vi "getVersion.vi"(8 "error in (no error)":errorcluster) -> (0 "error out":errorcluster, 2 "sbgComVersion":string, 3 "sbgMatLabVersion":string)   [LabVIEW 2011, in "sbgLabView.lvlib"]
uses:
  sbgLabView.lvlib
  sbgMatLab.dll
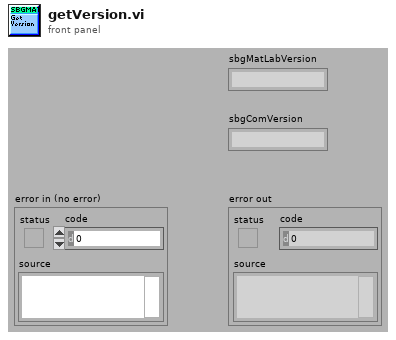
[diagram p1: front panel]
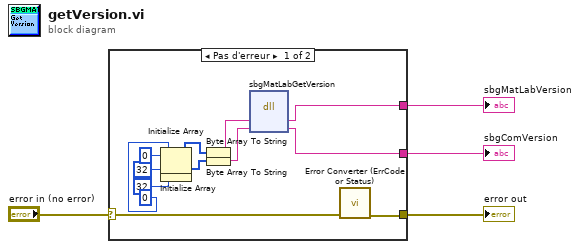
[diagram p0: block diagram]
diagram:
  n1 = case shown="Pas d'erreur" "error in (no error)" {
    selector: "error in (no error)" -> [w6 w17]
    tunnel: [w5 w17] -> w3
    tunnel: [w12 _] -> w2
    tunnel: [w7 _] -> w1
    frame No Error {
      n2 = Initialize Array(u8 0 ("element"), 32 ("dimension size")) -> (w16:u8[])
      n3 = Initialize Array(u8 0 ("element"), 32 ("dimension size")) -> (w11:u8[])
      n4 = Byte Array To String(unsigned byte array=w16) -> (string=w15:string)
      n5 = Byte Array To String(unsigned byte array=w11) -> (string=w10:string)
      n6 = dll-call lib="C:/SBG-Systems/remote/projects/software/projects/labviewExample/sbgLabView/sbgMatLab.*" fn="sbgMatLabGetVersion"("sbgMatLabVersion"=w15, "sbgComVersion"=w10) -> ("sbgMatLabVersion"=w12:string, "sbgComVersion"=w7:string)  [unwired: 4 in, 2 out]
      n7 = call "Error Converter (ErrCode or Status).vi"("error in (no error)"=w6) -> ("error out"=w5:errorcluster)  [unwired: 10 in]
    }
    frame Error {
    }
  }
  "sbgMatLabVersion" <- w2
  "sbgComVersion" <- w1
  "error out" <- w3
